vi "Create Reference.vi"   [LabVIEW 2015]
uses:
  <vilib>/Utility/miscctls.llb/LVPositionTypeDef.ctl
types:
  T1 = typedef "LVPositionTypeDef.ctl" = cluster{"Left":i32, "Top":i32}
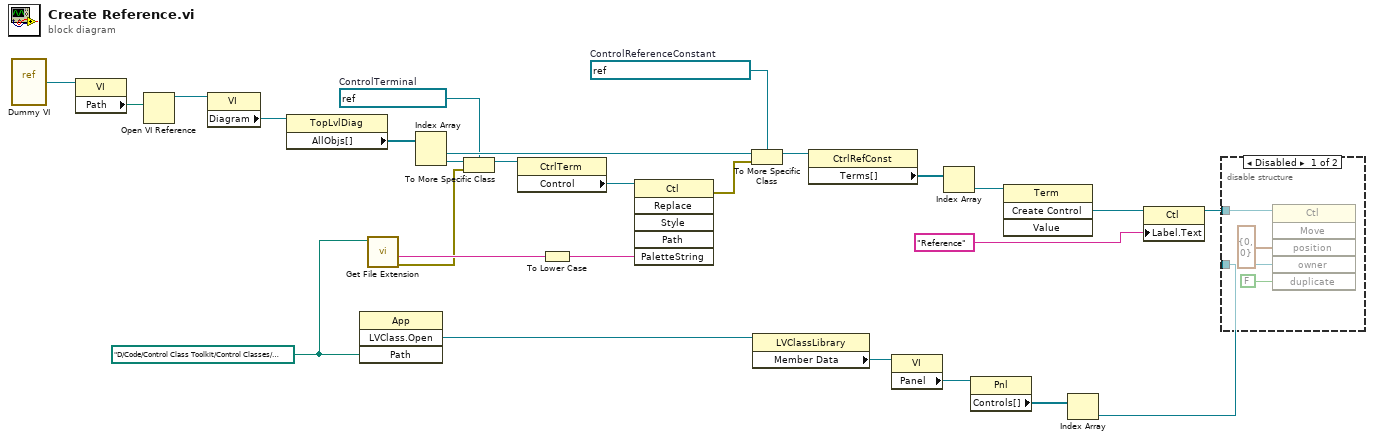
[diagram p0: block diagram]
diagram:
  w11 = refnum<vi> refnum  # ControlTerminal
  w9 = path "D:/Code/Control Class Toolkit/Control Classes/Boolean/Boolean.lvclass" ("Path")
  w23 = refnum<vi> refnum  # ControlReferenceConstant
  n1 = vi-ref "Dummy VI.vi"() -> (w4:refnum<vi>)
  n2 = property class="VI"(reference=w4) -> ("Path"=w3:path)  [unwired: 1 in, 2 out]
  n3 = Open VI Reference(vi path=w3) -> (vi reference=w27:refnum<vi>)  [unwired: 5 in, 1 out]
  n4 = property class="VI"(reference=w27) -> ("Diagram"=w26:refnum<vi>)  [unwired: 1 in, 2 out]
  n5 = property class="TopLvlDiag"(reference=w26) -> ("AllObjs[]"=w25:refnum<vi>[])  [unwired: 1 in, 2 out]
  n6 = invoke class="App" method="LVClass.Open"("Path"=w9) -> ("LVClass.Open"=w16:refnum<vi>)  [unwired: 3 in, 3 out]
  n7 = call <vilib>:"Get File Extension.vi"("file"=w9) -> ("error out"=w2:errorcluster, "filename without extension"=w8:string)  [unwired: 6 in, 3 out]
  n8 = Index Array(array=w25) -> (element #1=w24:refnum<vi>, element #2=w6:refnum<vi>)  [unwired: 2 in]
  n9 = To More Specific Class(target class=w11, reference=w6, error in=w2) -> (specific class reference=w10:refnum<vi>)  [unwired: 1 out]
  n10 = property class="CtrlTerm"(reference=w10) -> ("Control"=w5:refnum<vi>)  [unwired: 1 in, 2 out]
  n11 = To Lower Case(string=w8) -> (all lower case string=w1:string)
  n12 = invoke class="Ctl" method="Replace"(reference=w5, "PaletteString"=w1) -> (error out=w7:errorcluster)  [unwired: 4 in, 5 out]
  n13 = To More Specific Class(target class=w23, reference=w24, error in=w7) -> (specific class reference=w22:refnum<vi>)  [unwired: 1 out]
  n14 = property class="LVClassLibrary"(reference=w16) -> ("Member Data"=w15:refnum<vi>)  [unwired: 1 in, 2 out]
  n15 = property class="CtrlRefConst"(reference=w22) -> ("Terms[]"=w21:refnum<vi>[])  [unwired: 1 in, 2 out]
  n16 = property class="VI"(reference=w15) -> ("Panel"=w14:refnum<vi>)  [unwired: 1 in, 2 out]
  n17 = Index Array(array=w21) -> (element=w20:refnum<vi>)  [unwired: 1 in]
  n18 = property class="Pnl"(reference=w14) -> ("Controls[]"=w13:refnum<vi>[])  [unwired: 1 in, 2 out]
  n19 = invoke class="Term" method="Create Control"(reference=w20) -> ("Create Control"=w19:refnum<vi>)  [unwired: 3 in, 3 out]
  n20 = Index Array(array=w13) -> (element=w12:refnum<vi>)  [unwired: 1 in]
  n21 = property class="Ctl"(reference=w19, "Label.Text"="Reference") -> (reference out=w17:refnum<vi>)  [unwired: 1 in, 1 out]
  n22 = disable-structure shown="Disabled" {
    disable-tunnel: w17 -> [w31 _]
    disable-tunnel: w12 -> [w30 _]
    frame Disabled {
      n23 = invoke class="Ctl" method="Move"(reference=w31, "position"=T1 {"Left"=0, "Top"=0}, "owner"=w30, "duplicate"=FALSE ("Duplicate? (F)")) -> ()  [unwired: 2 in, 6 out]
    }
    frame Enabled {
    }
  }
